vi "create_LS372_Data_header.vi"() -> (3 "String":string)   [LabVIEW 2016]
uses:
  Instrument_Setup.vi
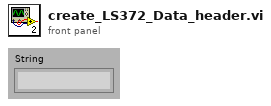
[diagram p1: front panel]
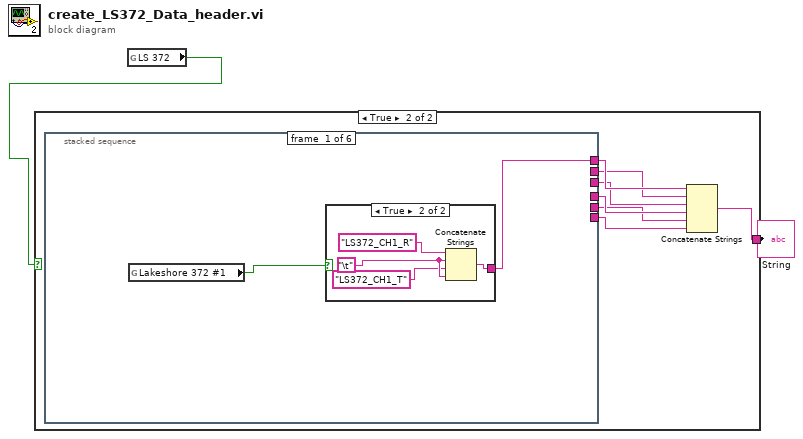
[diagram p0: block diagram]
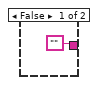
[diagram p2: hidden frame]
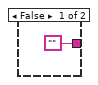
[diagram p3: hidden frame]
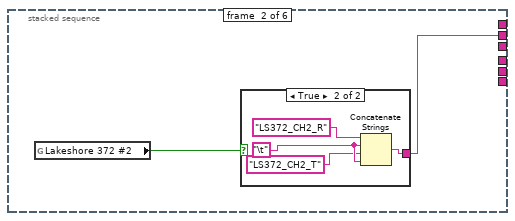
[diagram p4: hidden frame]
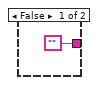
[diagram p5: hidden frame]
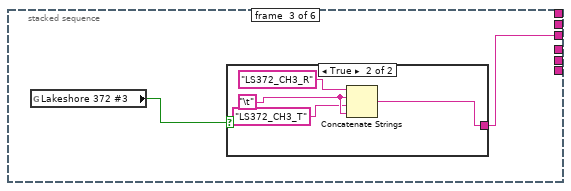
[diagram p6: hidden frame]
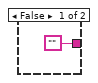
[diagram p7: hidden frame]
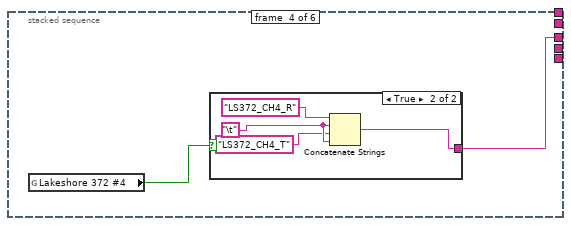
[diagram p8: hidden frame]
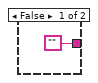
[diagram p9: hidden frame]
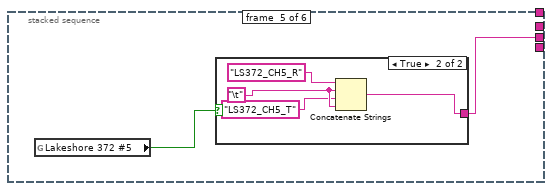
[diagram p10: hidden frame]
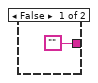
[diagram p11: hidden frame]
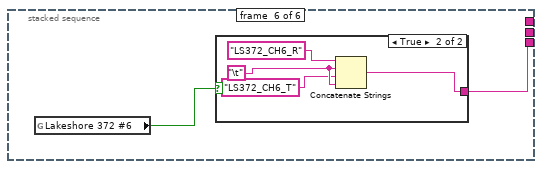
[diagram p12: hidden frame]
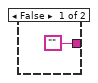
[diagram p13: hidden frame]
diagram:
  n1 = global read "Instrument_Setup.vi" "LS 372"() -> (w1:bool)
  n2 = case shown="True" w1 {
    tunnel: ["" w4] -> w2
    frame False {
    }
    frame True {
      n3 = stacked-sequence {
        tunnel: [w11 _ _ _ _ _] -> w10
        tunnel: [_ w18 _ _ _ _] -> w9
        tunnel: [_ _ w25 _ _ _] -> w8
        tunnel: [_ _ _ w32 _ _] -> w7
        tunnel: [_ _ _ _ w39 _] -> w6
        tunnel: [_ _ _ _ _ w46] -> w5
        frame #0 {
          n4 = global read "Instrument_Setup.vi" "Lakeshore 372 #1"() -> (w12:bool)
          n5 = case shown="True" w12 {
            tunnel: ["" w17] -> w11
            frame False {
            }
            frame True {
              w15 = "\t"
              n6 = Concatenate Strings("LS372_CH1_R", w15, "LS372_CH1_T", w15) -> (w17:string)
            }
          }
        }
        frame #1 {
          n7 = global read "Instrument_Setup.vi" "Lakeshore 372 #2"() -> (w19:bool)
          n8 = case shown="True" w19 {
            tunnel: ["" w24] -> w18
            frame False {
            }
            frame True {
              w22 = "\t"
              n9 = Concatenate Strings("LS372_CH2_R", w22, "LS372_CH2_T", w22) -> (w24:string)
            }
          }
        }
        frame #2 {
          n10 = global read "Instrument_Setup.vi" "Lakeshore 372 #3"() -> (w26:bool)
          n11 = case shown="True" w26 {
            tunnel: ["" w28] -> w25
            frame False {
            }
            frame True {
              w30 = "\t"
              n12 = Concatenate Strings("LS372_CH3_R", w30, "LS372_CH3_T", w30) -> (w28:string)
            }
          }
        }
        frame #3 {
          n13 = global read "Instrument_Setup.vi" "Lakeshore 372 #4"() -> (w33:bool)
          n14 = case shown="True" w33 {
            tunnel: ["" w35] -> w32
            frame False {
            }
            frame True {
              w37 = "\t"
              n15 = Concatenate Strings("LS372_CH4_R", w37, "LS372_CH4_T", w37) -> (w35:string)
            }
          }
        }
        frame #4 {
          n16 = global read "Instrument_Setup.vi" "Lakeshore 372 #5"() -> (w40:bool)
          n17 = case shown="True" w40 {
            tunnel: ["" w42] -> w39
            frame False {
            }
            frame True {
              w44 = "\t"
              n18 = Concatenate Strings("LS372_CH5_R", w44, "LS372_CH5_T", w44) -> (w42:string)
            }
          }
        }
        frame #5 {
          n19 = global read "Instrument_Setup.vi" "Lakeshore 372 #6"() -> (w47:bool)
          n20 = case shown="True" w47 {
            tunnel: ["" w49] -> w46
            frame False {
            }
            frame True {
              w51 = "\t"
              n21 = Concatenate Strings("LS372_CH6_R", w51, "LS372_CH6_T", w51) -> (w49:string)
            }
          }
        }
      }
      n22 = Concatenate Strings(w10, w9, w8, w7, w6, w5) -> (w4:string)
    }
  }
  "String" <- w2
